vi "OAT Verify Resampled Signal (Multi Channels).vi"(8 "error in (no error)":errorcluster, 11 "resampled signal":cluster{"r0":dbl, "dr":dbl, "Y":dbl[]}[](array[cluster]) {"r0" format="%.2p"; "dr" format="%.2p"; "Y" format="%.2f"}) -> (0 "error out":errorcluster, 2 "empty signal":bool, 3 "resampled signal out":cluster{"r0":dbl, "dr":dbl, "Y":dbl[]}[](array[cluster]))   [LabVIEW 2017, in "SoundVib_Resampling.lvlib"]
uses:
  <vilib>/addons/Sound and Vibration/Order Analysis/Resample Order Tracking/SoundVib_Resampling.lvlib
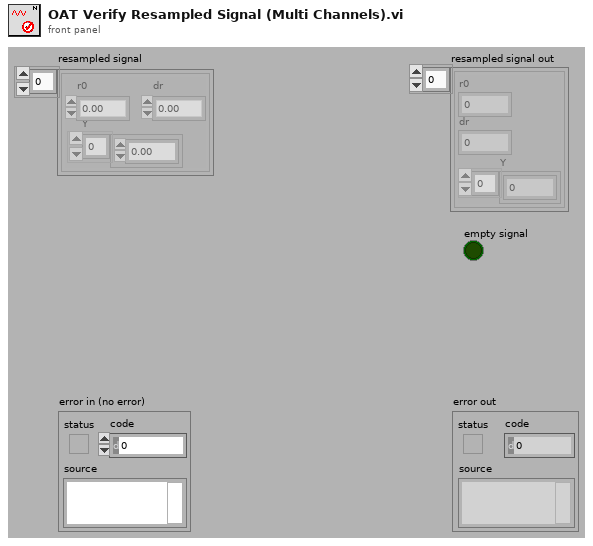
[diagram p1: front panel]
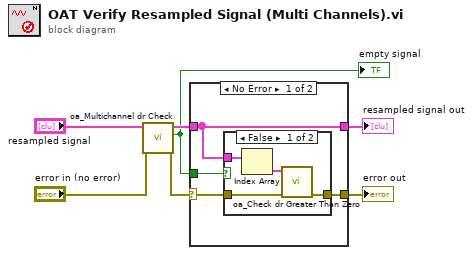
[diagram p0: block diagram]
diagram:
  n1 = call <vilib>:"oa_Multichannel dr Check.vi"("error in (no error)"="error in (no error)", "resampled signal in"="resampled signal") -> ("error out"=w2:errorcluster, "empty signal"=w1:bool, "resampled signal out"=w4:cluster{"r0":dbl, "dr":dbl, "Y":dbl[]}[])  [unwired: 7 in]
  "empty signal" <- w1
  n2 = case shown="No Error" w2 {
    selector: w2 -> [w10 w17]
    tunnel: [w11 w17] -> w7
    tunnel: w4 -> [w9 w18]
    tunnel: [w9 w18] -> w6
    tunnel: w1 -> [w8 _]
    frame No Error {
      n3 = case shown="False" w8 {
        tunnel: [w15 w16] -> w11
        tunnel: w10 -> [w14 w16]
        tunnel: w9 -> [w12 _]
        frame False {
          n4 = Index Array(array=w12) -> (element=w13:cluster{"r0":dbl, "dr":dbl, "Y":dbl[]})  [unwired: 1 in]
          n5 = call <vilib>:"oa_Check dr Greater Than Zero.vi"("error in (no error)"=w14, "resampled signal"=w13) -> ("error out"=w15:errorcluster)  [unwired: 8 in, 1 out]
        }
        frame True {
        }
      }
    }
    frame Error {
    }
  }
  "error out" <- w7
  "resampled signal out" <- w6
